vi "LVClass_Camera Disconnect.vi"(0 "Camera in":refnum<class "Camera.lvclass">, 11 "error in (no error)":errorcluster) -> (4 "Camera out":refnum<class "Camera.lvclass">, 15 "error out":errorcluster)   [LabVIEW 2020, in "Camera.lvclass"]
doc: "Close connection to the device.\n\n<B>CameraIn</B> : Camera object.\n<B>CameraOut</B> : Camera object."
uses:
  Camera.lvclass
  Camera.lvclass/Camera.ctl
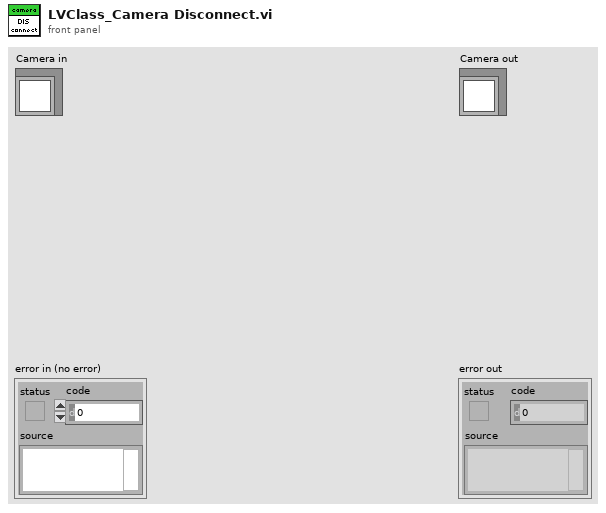
[diagram p1: front panel]
types:
  T1 = typedef "ClassID.ctl" = i64
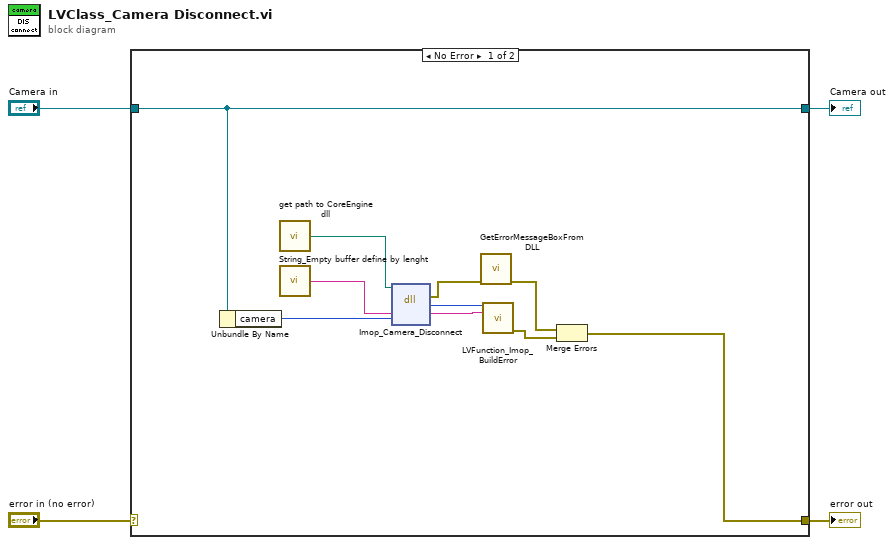
[diagram p0: block diagram]
diagram:
  n1 = case shown="No Error" "error in (no error)" {
    selector: "error in (no error)" -> [_ w16]
    tunnel: [w5 w16] -> w3
    tunnel: [w6 w15] -> w1
    tunnel: "Camera in" -> [w6 w15]
    frame No Error {
      n2 = Unbundle By Name(w6) -> ("camera"=w9:T1)
      n3 = call "get path to CoreEngine dll.vi"() -> ("path to c_interface_vc100.dll"=w11:path)  [unwired: 12 in, 3 out]
      n4 = call "String_Empty buffer define by lenght.vi"() -> ("Empty buffer"=w14:string)  [unwired: 1 in]
      n5 = dll-call lib="D:/soft/HASO_v3/SVN_trunk/ImOpCoreEngine4_LV2011/DLLs/c_interface_vc100.dll" fn="Imop_Camera_Disconnect"(path in=w11, "message"=w14, "objet"=w9) -> (error out=w10:errorcluster, "return type"=w12:i32, "message"=w13:string)  [unwired: 3 in, 1 out]
      n6 = call "GetErrorMessageBoxFromDLL.vi"("error IN"=w10) -> ("error OUT"=w8:errorcluster)  [unwired: 10 in]
      n7 = call "LVFunction_Imop_BuildError.vi"("code"=w12, "String to Prepend to source (\"\")"=w13) -> ("error out"=w7:errorcluster)  [unwired: 13 in]
      n8 = Merge Errors(w8, w7) -> (w5:errorcluster)
    }
    frame Error {
    }
  }
  "error out" <- w3
  "Camera out" <- w1
